vi "StopCond to string.vi"(11 "StopCond param":T1(ring)) -> (3 "String":string)   [LabVIEW 2019, in "STAV lib.lvlib"]
uses:
  STAV lib.lvlib
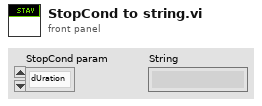
[diagram p1: front panel]
types:
  T1 = enum16{"dUration", "dIstance", "Position", "force Greater", "force Smaller", "Break", "keep Force"}
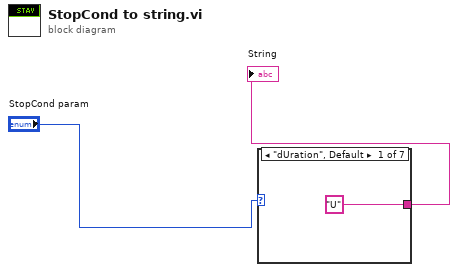
[diagram p0: block diagram]
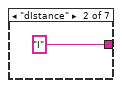
[diagram p2: hidden frame]
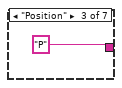
[diagram p3: hidden frame]
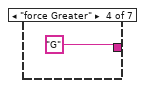
[diagram p4: hidden frame]
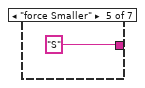
[diagram p5: hidden frame]
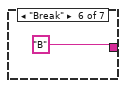
[diagram p6: hidden frame]
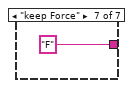
[diagram p7: hidden frame]
diagram:
  n1 = case shown="\"dUration\", Default" "StopCond param" {
    tunnel: ["U" "I" "P" "G" "S" "B" "F"] -> w2
    frame "dUration", Default {
    }
    frame "dIstance" {
    }
    frame "Position" {
    }
    frame "force Greater" {
    }
    frame "force Smaller" {
    }
    frame "Break" {
    }
    frame "keep Force" {
    }
  }
  "String" <- w2
